vi "NF WF1973_74 OUTP Am.vi"(6 "Read(F)":bool, 8 "error in (no error)":errorcluster caption="Error IN", 9 "AM type(Sync)":u16(ring) items=["Sync", "Msync", "Mfctn"], 10 "Ch(Ch1)":bool, 11 "VISAsession":refnum<visa-resource-name>) -> (0 "error out":errorcluster caption="Error OUT", 2 "Query AM type":string, 3 "CopyVISAsession":refnum<visa-resource-name>)   [LabVIEW 2010]
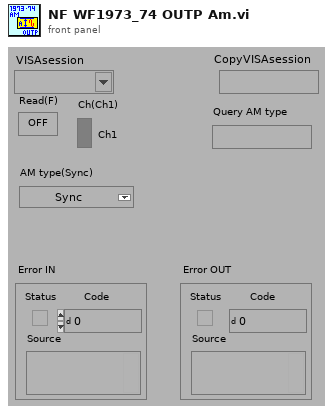
[diagram p1: front panel]
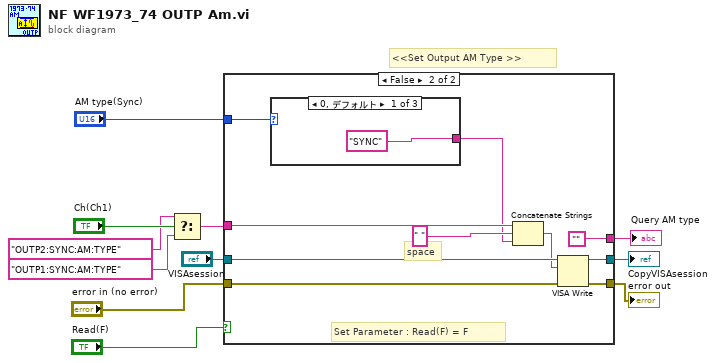
[diagram p0: block diagram]
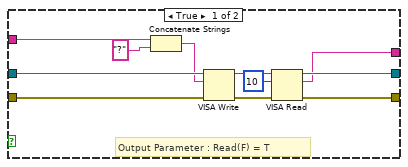
[diagram p2: hidden frame]
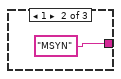
[diagram p3: hidden frame]
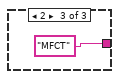
[diagram p4: hidden frame]
diagram:
  # "<<Set Output AM Type >>"
  n1 = Select(t="OUTP2:SYNC:AM:TYPE" ("文字列"), s="Ch(Ch1)", f="OUTP1:SYNC:AM:TYPE" ("文字列")) -> (s? t:f=w4:string)
  n2 = case shown="FALSE" "Read(F)" {
    tunnel: "VISAsession" -> [w22 w32]
    tunnel: [w19 w30] -> w10
    tunnel: [w18 w31] -> w9
    tunnel: "error in (no error)" -> [w17 w26]
    tunnel: w4 -> [w15 w27]
    tunnel: [w12 ""] -> w6
    tunnel: "AM type(Sync)" -> [_ w25]
    frame True {
      # "Output Parameter : Read(F) = T"
      n3 = Concatenate Strings(w15, "?" ("形式文字列")) -> (w13:string)
      n4 = VISA Write(VISA resource name=w22, write buffer=w13, error in (no error)=w17) -> (VISA resource name out=w20:refnum<visa-resource-name>, error out=w21:errorcluster)  [unwired: 1 out]
      n5 = VISA Read(VISA resource name=w20, byte count=u32 10 ("バイトカウント（0）"), error in (no error)=w21) -> (VISA resource name out=w19:refnum<visa-resource-name>, read buffer=w12:string, error out=w18:errorcluster)  [unwired: 1 out]
    }
    frame False {
      # "space"
      # "Set Parameter : Read(F) = F"
      n6 = case shown="0, デフォルト" w25 {
        tunnel: ["SYNC" ("文字列") "MSYN" ("文字列") "MFCT" ("文字列")] -> w24
        frame 0, Default {
        }
        frame 1 {
        }
        frame 2 {
        }
      }
      n7 = Concatenate Strings(w27, " ", w24) -> (w29:string)
      n8 = VISA Write(VISA resource name=w32, write buffer=w29, error in (no error)=w26) -> (VISA resource name out=w30:refnum<visa-resource-name>, error out=w31:errorcluster)  [unwired: 1 out]
    }
  }
  "error out" <- w9
  "CopyVISAsession" <- w10
  "Query AM type" <- w6
